vi "Find Event Frame.vi"(9 "Broadcast?":bool, 10 "VI in":refnum<vi>, 11 "Application Instance":refnum<vi>) -> (0 "error out":errorcluster)   [LabVIEW 2019, in "Panther Dashboard.lvlib"]
uses:
  Panther Dashboard.lvlib
  <vilib>/Utility/traverseref.llb/TRef TravTarget.ctl
  <vilib>/Utility/traverseref.llb/VI Scripting - Traverse.lvlib
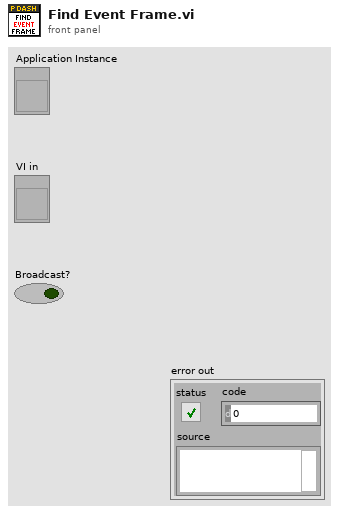
[diagram p1: front panel]
types:
  T1 = typedef "TRef TravTarget.ctl" = enum16{"FP", "BD", "Other"}
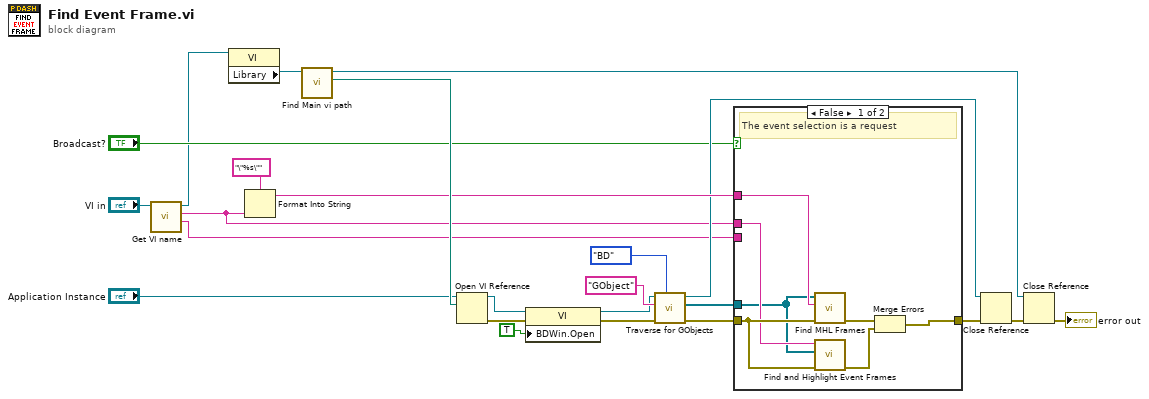
[diagram p0: block diagram]
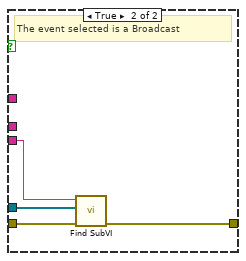
[diagram p2: hidden frame]
diagram:
  n1 = call "Get VI name.vi"("VI in"="VI in") -> ("Full Vi Name"=w5:string, "Plain Name"=w3:string, "VI out"=w1:refnum<vi>)  [unwired: 8 in]
  n2 = property class="VI"(reference=w1) -> ("Library"=w2:refnum<vi>)  [unwired: 1 in, 2 out]
  n3 = Format Into String(format string="\"%s\"", w3) -> (resulting string=w13:string)  [unwired: 2 in, 1 out]
  n4 = call "Find Main vi path.vi"("Library"=w2) -> ("Main vi Path"=w17:path, "Library out"=w15:refnum<vi>)  [unwired: 9 in]
  n5 = Open VI Reference(application reference (local)="Application Instance", vi path=w17) -> (vi reference=w16:refnum<vi>, error out=w24:errorcluster)  [unwired: 4 in]
  n6 = property class="VI"(reference=w16, error in=w24, "BDWin.Open"=TRUE ("Block Diagram Window:Open")) -> (reference out=w9:refnum<vi>, error out=w23:errorcluster)
  n7 = call <vilib>:"Traverse for GObjects.vi"("Traverse Target"=TRef_TravTarget."BD", "error in (no error)"=w23, "Class Name"="GObject", "VI Refnum"=w9) -> ("error out"=w22:errorcluster, "References"=w8:refnum<vi>[], "dup VI Refnum"=w7:refnum<vi>)  [unwired: 4 in, 1 out]
  n8 = case shown="False" "Broadcast?" {
    tunnel: w13 -> [w27 _]
    tunnel: w22 -> [w31 w35]
    tunnel: w8 -> [w25 w32]
    tunnel: w5 -> [_ w33]
    tunnel: w3 -> [w26 _]
    tunnel: [w29 w34] -> w20
    frame False {
      # "The event selection is a request"
      n9 = call "Find MHL Frames.vi"("error in"=w31, "Event"=w27, "References"=w25) -> ("error out"=w30:errorcluster)  [unwired: 8 in]
      n10 = call "Find and Highlight Event Frames.vi"("error in"=w31, "References"=w25, "Event Name"=w26) -> ("error out"=w28:errorcluster)  [unwired: 8 in]
      n11 = Merge Errors(w30, w28) -> (w29:errorcluster)
    }
    frame True {
      # "The event selected is a Broadcast"
      n12 = call "Find SubVI.vi"("error in"=w35, "References"=w32, "Full Vi Name"=w33) -> ("error out"=w34:errorcluster)  [unwired: 8 in]
    }
  }
  n13 = Close Reference(reference=w7, error in (no error)=w20) -> (error out=w19:errorcluster)
  n14 = Close Reference(reference=w15, error in (no error)=w19) -> (error out=→"error out":errorcluster)
